vi "Adjust Temperature.vi"(7 "System Status":enum16{"Heating", "Cooling", "Idle"}(ring)=enum."Cooling", 8 "error in (no error)":errorcluster, 10 "Setpoint (°F) in":dbl, 11 "Current Temperature (°F) in":dbl) -> (0 "error out":errorcluster, 1 "Equal Temps?":bool, 2 "Setpoint (°F) out":dbl, 3 "Current Temperature (°F) out":dbl)   [LabVIEW 2026]
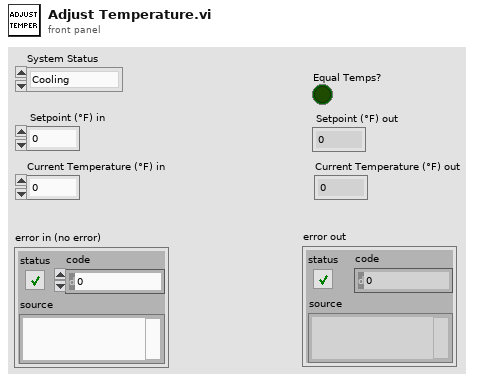
[diagram p1: front panel]
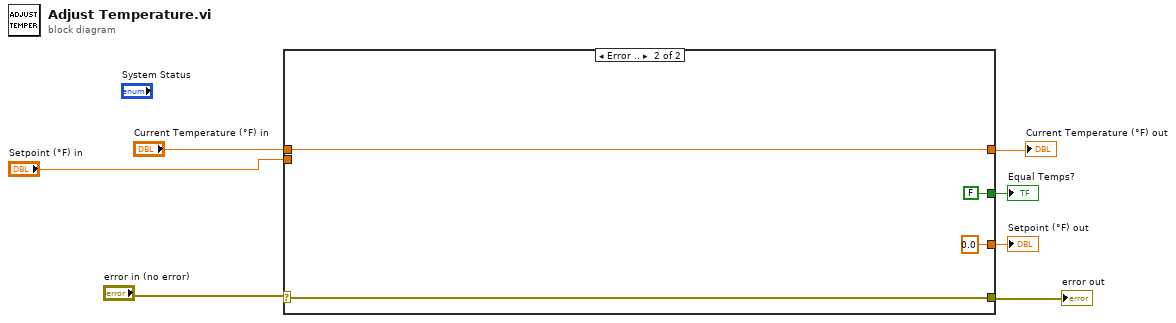
[diagram p0: block diagram]
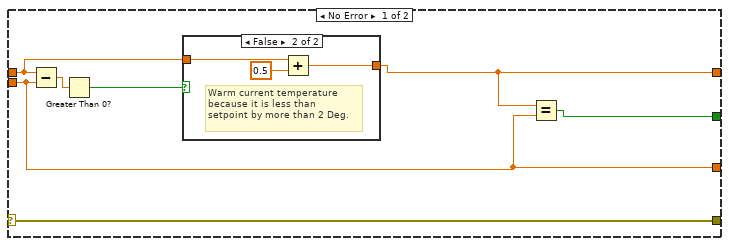
[diagram p2: hidden frame]
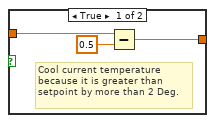
[diagram p3: hidden frame]
diagram:
  n1 = case shown="Error .." "error in (no error)" {
    selector: "error in (no error)" -> [w14 w24]
    tunnel: "Setpoint (°F) in" -> [w8 _]
    tunnel: "Current Temperature (°F) in" -> [w11 w23]
    tunnel: [w14 w24] -> w4
    tunnel: [w10 w23] -> w3
    tunnel: [w9 FALSE] -> w2
    tunnel: [w8 0.0 ("Setpoint (°F) in")] -> w1
    frame No Error {
      n2 = Subtract(x=w11, y=w8) -> (x-y=w13:dbl)
      n3 = Greater Than 0?(x=w13) -> (x > 0?=w12:bool)
      n4 = case shown="False" w12 {
        tunnel: w11 -> [w17 w20]
        tunnel: [w15 w18] -> w10
        frame True {
          # "Cool current temperature\nbecause it is greater than\nsetpoint by more than 2 Deg."
          n5 = Subtract(x=w17, y=0.5) -> (x-y=w15:dbl)
        }
        frame False {
          # "Warm current temperature\nbecause it is less than\nsetpoint by more than 2 Deg."
          n6 = Add(x=w20, y=0.5) -> (x+y=w18:dbl)
        }
      }
      n7 = Equal?(x=w10, y=w8) -> (x = y?=w9:bool)
    }
    frame Error {
    }
  }
  "error out" <- w4
  "Current Temperature (°F) out" <- w3
  "Equal Temps?" <- w2
  "Setpoint (°F) out" <- w1
